vi "Final.vi"() -> ()   [LabVIEW 2020]
uses:
  pattern attempt/simon/simon_colors.ctl
panel:
  out "red":bool
  out "yellow":bool
  out "green":bool
  out "blue":bool
  out "Score":i32
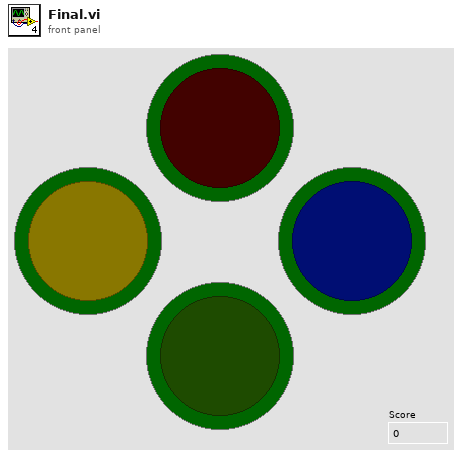
[diagram p1: front panel]
types:
  T1 = typedef "simon_colors.ctl" = enum16{"red", "green", "yellow", "blue"}
  T2 = enum16{"Left Button", "Center Button", "Right Button", "Window Close"}
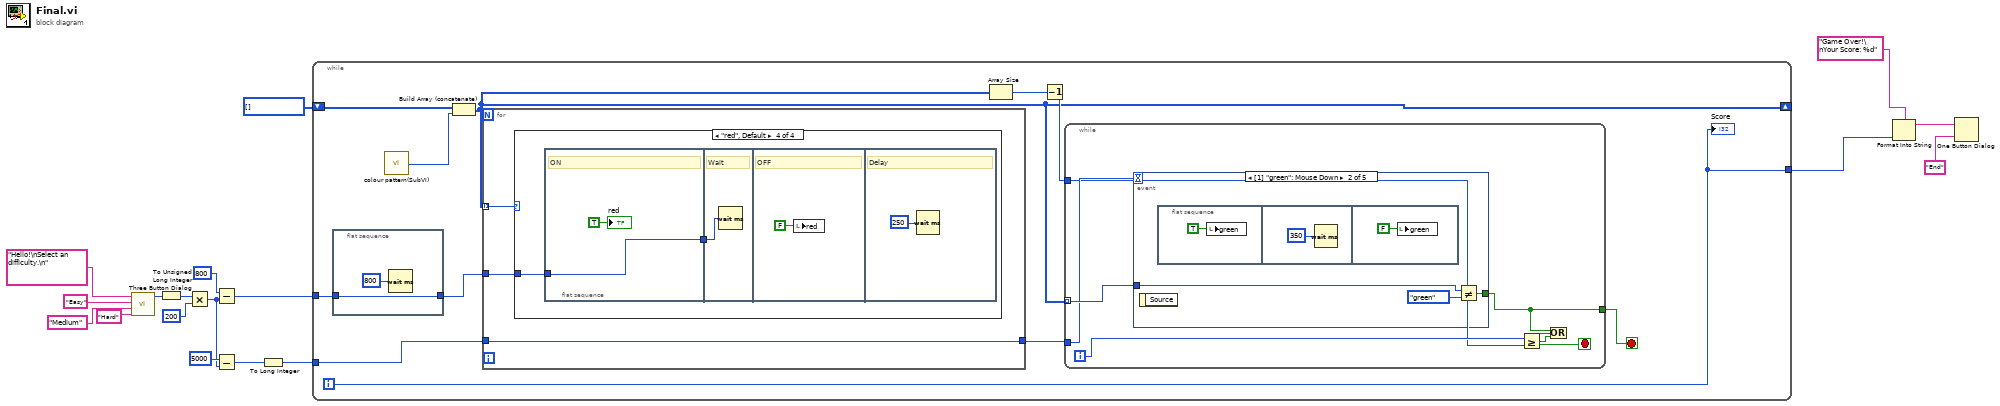
[diagram p0: block diagram]
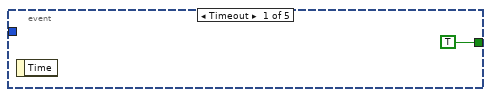
[diagram p2: hidden frame]
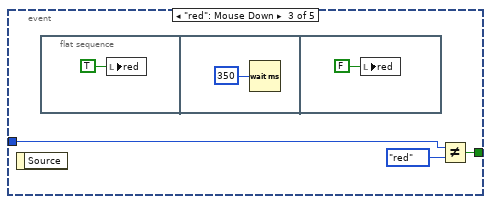
[diagram p3: hidden frame]
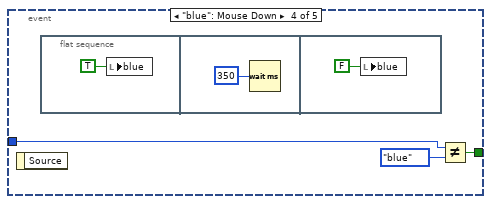
[diagram p4: hidden frame]
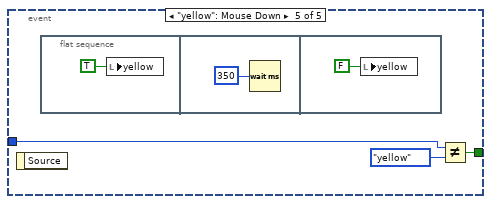
[diagram p5: hidden frame]
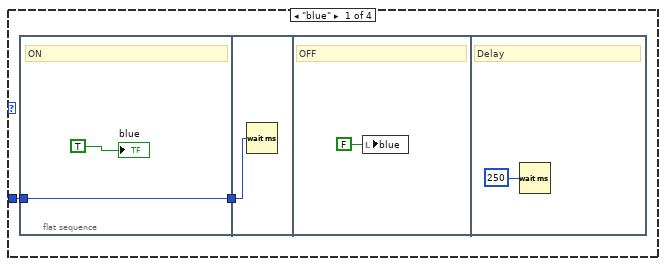
[diagram p6: hidden frame]
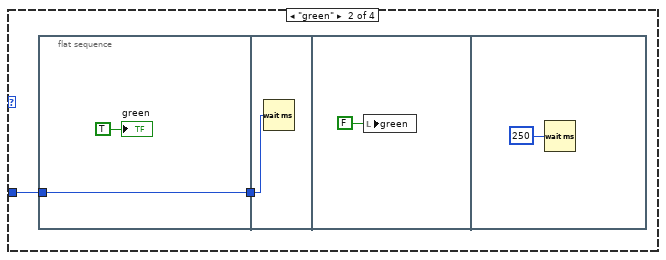
[diagram p7: hidden frame]
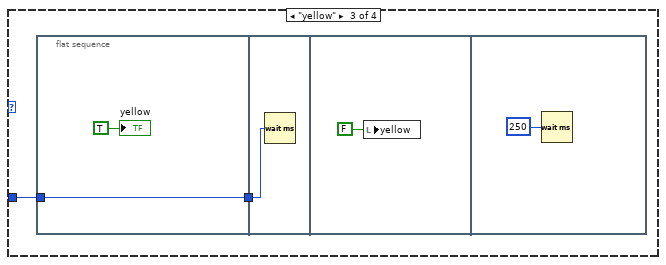
[diagram p8: hidden frame]
diagram:
  w16 = T1[] [] items=["red", "green", "yellow", "blue"]
  n1 = call <vilib>:"Three Button Dialog.vi"("Right Button Text (\"Cancel\")"="Hard" ("Right Button Text (\"Cancel\")"), "Center Button Text (\"No\")"="Medium" ("Center Button Text (\"No\")"), "Left Button Text (\"Yes\")"="Easy" ("Left Button Text (\"Yes\")"), "message"="Hello!\nSelect an difficulty.\n") -> ("Which Button?"=w9:T2)  [unwired: 7 in]
  n2 = To Unsigned Long Integer(number=w9) -> (unsigned 32bit integer=w4:u32)
  n3 = Multiply(x=w4, y=u32 200) -> (x*y=w1:u32)
  n4 = Subtract(x=u32 800 ("millisecond multiple"), y=w1) -> (x-y=w17:u32)
  n5 = Subtract(x=u32 5000, y=w1) -> (x-y=w12:u32)
  n6 = To Long Integer(number=w12) -> (32bit integer=w2:i32)
  n7 = while {
    shift-right: [w20] -> _
    shift-left: w16 -> [w28]
    tunnel: [w29] -> w18
    tunnel: w17 -> [w21]
    tunnel: w2 -> [w24]
    i -> [w29]
    stop <- w25 stop-if-true
    n8 = flat-sequence {
      tunnel: [w31] -> w22
      tunnel: w21 -> [w31]
      frame #0 {
        n9 = Wait (ms)(milliseconds to wait=u32 800 ("millisecond multiple")) -> ()  [unwired: 1 out]
      }
    }
    n10 = call "colour pattern(SubVI).vi"() -> ("Color Selected"=w19:T1)  [unwired: 1 in]
    n11 = Build Array (concatenate)(w28, w19) -> (w20:T1[])
    n12 = for {
      tunnel: w20 -> [w66] mode=indexing
      tunnel: w22 -> [w65]
      tunnel: [w64] -> w23
      tunnel: w24 -> [w64]
      n13 = case shown="\"red\", Default" w66 {
        tunnel: w65 -> [w68 w74 w81 w88]
        frame "blue" {
          n14 = flat-sequence {
            tunnel: w68 -> [w70]
            tunnel: [w70] -> w67
            tunnel: w67 -> [w71]
            frame #0 {
              # "ON"
              "blue" <- TRUE ("blue")
            }
            frame #1 {
              n15 = Wait (ms)(milliseconds to wait=w71) -> ()  [unwired: 1 out]
            }
            frame #2 {
              # "OFF"
              n16 = local write "blue"(FALSE ("blue")) -> ()
            }
            frame #3 {
              # "Delay"
              n17 = Wait (ms)(milliseconds to wait=u32 250 ("millisecond multiple")) -> ()  [unwired: 1 out]
            }
          }
        }
        frame "green" {
          n18 = flat-sequence {
            tunnel: w74 -> [w77]
            tunnel: [w77] -> w75
            tunnel: w75 -> [w78]
            frame #0 {
              "green" <- TRUE ("green")
            }
            frame #1 {
              n19 = Wait (ms)(milliseconds to wait=w78) -> ()  [unwired: 1 out]
            }
            frame #2 {
              n20 = local write "green"(FALSE ("green")) -> ()
            }
            frame #3 {
              n21 = Wait (ms)(milliseconds to wait=u32 250 ("millisecond multiple")) -> ()  [unwired: 1 out]
            }
          }
        }
        frame "yellow" {
          n22 = flat-sequence {
            tunnel: w81 -> [w84]
            tunnel: [w84] -> w82
            tunnel: w82 -> [w85]
            frame #0 {
              "yellow" <- TRUE ("yellow")
            }
            frame #1 {
              n23 = Wait (ms)(milliseconds to wait=w85) -> ()  [unwired: 1 out]
            }
            frame #2 {
              n24 = local write "yellow"(FALSE ("yellow")) -> ()
            }
            frame #3 {
              n25 = Wait (ms)(milliseconds to wait=u32 250 ("millisecond multiple")) -> ()  [unwired: 1 out]
            }
          }
        }
        frame "red", Default {
          n26 = flat-sequence {
            tunnel: w88 -> [w91]
            tunnel: [w91] -> w89
            tunnel: w89 -> [w92]
            frame #0 {
              # "ON"
              "red" <- TRUE ("red")
            }
            frame #1 {
              # "Wait"
              n27 = Wait (ms)(milliseconds to wait=w92) -> ()  [unwired: 1 out]
            }
            frame #2 {
              # "OFF"
              n28 = local write "red"(FALSE ("red")) -> ()
            }
            frame #3 {
              # "Delay"
              n29 = Wait (ms)(milliseconds to wait=u32 250 ("millisecond multiple")) -> ()  [unwired: 1 out]
            }
          }
        }
      }
    }
    n30 = Array Size(array=w20) -> (size(s)=w27:i32)
    n31 = Decrement(x=w27) -> (x-1=w26:i32)
    n32 = while {
      tunnel: w20 -> [w38] mode=indexing
      tunnel: [w36] -> w25
      tunnel: w23 -> [w37]
      tunnel: w26 -> [w34]
      i -> [w35]
      stop <- w32 stop-if-true
      n33 = event shown="[1] \"green\": Mouse Down" {
        selector: _ -> [_ _ _ _ _]
        dyn-events: _ -> [_ _ _ _ _]
        timeout: w37 -> [_ _ _ _ _]
        tunnel: w38 -> [_ w41 w47 w53 w60]
        tunnel: [TRUE w40 w46 w52 w58] -> w36
        event Timeout {
          n34 = event-data() -> ()  [unwired: 1 in, 1 out]
        }
        event "green": Mouse Down {
          n35 = event-data() -> ()  [unwired: 1 in, 1 out]
          n36 = flat-sequence {
            frame #0 {
              n37 = local write "green"(TRUE ("red")) -> ()
            }
            frame #1 {
              n38 = Wait (ms)(milliseconds to wait=u32 350) -> ()  [unwired: 1 out]
            }
            frame #2 {
              n39 = local write "green"(FALSE ("red")) -> ()
            }
          }
          n40 = Not Equal?(x=w41, y=simon_colors."green" ("Color Selected")) -> (x != y?=w40:bool)
        }
        event "red": Mouse Down {
          n41 = event-data() -> ()  [unwired: 1 in, 1 out]
          n42 = flat-sequence {
            frame #0 {
              n43 = local write "red"(TRUE ("red")) -> ()
            }
            frame #1 {
              n44 = Wait (ms)(milliseconds to wait=u32 350) -> ()  [unwired: 1 out]
            }
            frame #2 {
              n45 = local write "red"(FALSE ("red")) -> ()
            }
          }
          n46 = Not Equal?(x=w47, y=simon_colors."red" ("Color Selected")) -> (x != y?=w46:bool)
        }
        event "blue": Mouse Down {
          n47 = event-data() -> ()  [unwired: 1 in, 1 out]
          n48 = flat-sequence {
            frame #0 {
              n49 = local write "blue"(TRUE ("red")) -> ()
            }
            frame #1 {
              n50 = Wait (ms)(milliseconds to wait=u32 350) -> ()  [unwired: 1 out]
            }
            frame #2 {
              n51 = local write "blue"(FALSE ("red")) -> ()
            }
          }
          n52 = Not Equal?(x=w53, y=simon_colors."blue" ("Color Selected")) -> (x != y?=w52:bool)
        }
        event "yellow": Mouse Down {
          n53 = event-data() -> ()  [unwired: 1 in, 1 out]
          n54 = flat-sequence {
            frame #0 {
              n55 = local write "yellow"(TRUE ("red")) -> ()
            }
            frame #1 {
              n56 = Wait (ms)(milliseconds to wait=u32 350) -> ()  [unwired: 1 out]
            }
            frame #2 {
              n57 = local write "yellow"(FALSE ("red")) -> ()
            }
          }
          n58 = Not Equal?(x=w60, y=simon_colors."yellow" ("Color Selected")) -> (x != y?=w58:bool)
        }
      }
      n59 = Greater Or Equal?(x=w35, y=w34) -> (x >= y?=w33:bool)
      n60 = Or(x=w36, y=w33) -> (x .or. y?=w32:bool)
    }
    "Score" <- w29
  }
  n61 = Format Into String(format string="Game Over!\nYour Score: %d" ("initial string"), w18) -> (resulting string=w13:string)  [unwired: 2 in, 1 out]
  n62 = One Button Dialog(message=w13, button name ("OK")="End") -> ()  [unwired: 1 out]
